vi "Filter Set Averaging Frame Count.vi"(11 "frames":i32) -> (3 "function return":u32)   [LabVIEW 2018, in "Copy of Andor SDK.lvlib"]
doc: "EXPNETTYPE unsigned int WINAPI Filter_SetAveragingFrameCount(int frames);"
uses:
  Copy of Andor SDK.lvlib
  <userlib>/Andor SDK/ATMCD32D.dll
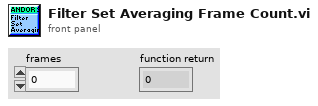
[diagram p1: front panel]
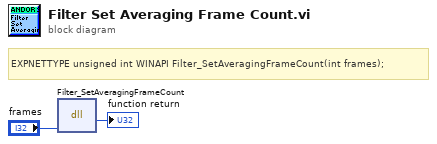
[diagram p0: block diagram]
diagram:
  # "EXPNETTYPE unsigned int WINAPI Filter_SetAveragingFrameCount(int frames);"
  n1 = dll-call lib="C:/Program Files (x86)/National Instruments/LabVIEW 2018/user.lib/Andor SDK/ATMCD32D.*" fn="Filter_SetAveragingFrameCount"("frames"="frames") -> (→"function return":u32)  [unwired: 4 in, 2 out]
